vi "Notify Counter Branch.vi"(8 "EventLog":refnum<class "abs_EventLog.lvclass">, 9 "Time (ms)":u32=40, 10 "Blackboard Group":string="B", 11 "Blackboard in":refnum<class "Blackboard.lvclass">) -> (3 "bt_Node out":refnum<class "bt_Node.lvclass">)   [LabVIEW 2021]
uses:
  Blackboard/Blackboard.lvclass
  Support/Nodes/abs_Node/bt_Node.lvclass
  Support/Nodes/Decorators/Repeater/Support/Finish On - Type.ctl
  Blackboard/Blackboard.lvclass/Blackboard.ctl
  Support/Nodes/Leaves/abs_Type Leaf/abs_Type Leaf.lvclass/abs_Type Leaf.ctl
  Blackboard/Get Value Type/Get I32.vi
  Blackboard/Support/Index Group.vi
  Blackboard/Support/Index Tags.vi
  Support/Nodes/Leaves/abs_Type Leaf/Properties/Write Value Class.vi
  <vilib>/TSA/Abstract Data Classes/Abs_Types/I32 Integer/Abs_I32 Integer.lvclass
  C:/Program Files (x86)/National Instruments/LabVIEW 2021/vi.lib/TSA/Abstract Data Classes/Abs_Types/Value/Abs_Value.lvclass
  C:/Program Files (x86)/National Instruments/LabVIEW 2021/vi.lib/TSA/Abstract Data Classes/Abs_Types/Numeric/Abs_Numeric.lvclass
  <vilib>/TSA/Omni-Bus/Local Bus/Support/I32/Local Bus_I32.lvclass
  Support/Nodes/Leaves/Test Boolean/Test Abs_Boolean.lvclass
  C:/Users/timst/Documents/Repositories/LV_Behaviour_Tree/Source/Support/Nodes/abs_Node/bt_Node.lvclass
  C:/Users/timst/Documents/Repositories/LV_Behaviour_Tree/Source/Support/Nodes/Leaves/abs_Type Leaf/abs_Type Leaf.lvclass
  <vilib>/TSA/Abstract Data Classes/Abs_Types/Boolean/Abs_Boolean.lvclass
  C:/Program Files (x86)/National Instruments/LabVIEW 2021/vi.lib/TSA/Abstract Data Classes/Abs_Types/Type/Abs_Type.lvclass
  <vilib>/TSA/Omni-Bus/Local Bus/Support/Initialise DVR's.vi
  <vilib>/TSA/Abstract Data Classes/Abs_Types/Value/Abs_Value.lvclass
  <vilib>/TSA/Abstract Data Classes/Abs_Types/Type/Abs_Type.lvclass
  <vilib>/TSA/Omni-Bus/Local Bus/Support/DBL/Local Bus_DBL.lvclass
  <vilib>/TSA/Omni-Bus/Local Bus/Support/SGL/Local Bus_SGL.lvclass
  <vilib>/TSA/Omni-Bus/Local Bus/Support/EXT/Local Bus_EXT.lvclass
  <vilib>/TSA/Omni-Bus/Local Bus/Support/Bool/Local Bus_Boolean.lvclass
  <vilib>/TSA/Omni-Bus/Local Bus/Support/STR/Local Bus_String.lvclass
  <vilib>/TSA/Omni-Bus/Local Bus/Support/Variant/Local Bus_Variant.lvclass
  <vilib>/TSA/Omni-Bus/Local Bus/Support/WFM/Local Bus_Waveform.lvclass
  <vilib>/TSA/Omni-Bus/Local Bus/Support/Time/Local Bus_Time.lvclass
  <vilib>/TSA/Omni-Bus/Local Bus/Support/U8/Local Bus_U8.lvclass
  <vilib>/TSA/Omni-Bus/Local Bus/Support/U16/Local Bus_U16.lvclass
  <vilib>/TSA/Omni-Bus/Local Bus/Support/U32/Local Bus_U32.lvclass
  <vilib>/TSA/Omni-Bus/Local Bus/Support/U64/Local Bus_U64.lvclass
  <vilib>/TSA/Omni-Bus/Local Bus/Support/I8/Local Bus_I8.lvclass
  <vilib>/TSA/Omni-Bus/Local Bus/Support/I16/Local Bus_I16.lvclass
  <vilib>/TSA/Omni-Bus/Local Bus/Support/I64/Local Bus_I64.lvclass
  <vilib>/TSA/Omni-Bus/Local Bus/Support/CSGL/Local Bus_CSGL.lvclass
  <vilib>/TSA/Omni-Bus/Local Bus/Support/CDBL/Local Bus_CDBL.lvclass
  <vilib>/TSA/Omni-Bus/Local Bus/Support/CEXT/Local Bus_CEXT.lvclass
  <vilib>/TSA/Omni-Bus/Local Bus/Support/Type/Local Bus_Type.lvclass
  <vilib>/TSA/Abstract Data Classes/Functions/Compare/Support/Greater Equal/I32/Method.vi
  <vilib>/TSA/Abstract Data Classes/Functions/Math/Support/Increment/I32/Method.vi
  <vilib>/TSA/Abstract Data Classes/Constants/Support/I32/I32.vi
  BT.lvlib
  Support/Nodes/Decorators/Repeater/bt_Repeater.lvclass
  C:/Program Files (x86)/National Instruments/LabVIEW 2021/vi.lib/TSA/Abstract Data Classes/Abs_Types/Integer/Abs_Integer.lvclass
  C:/Program Files (x86)/National Instruments/LabVIEW 2021/vi.lib/TSA/Abstract Data Classes/Abs_Types/I32 Integer/Abs_I32 Integer.lvclass
  <vilib>/TSA/Abstract Data Classes/Functions/Compare/Support/Greater Equal/I32/Greater Equal_I32.lvclass
  <vilib>/TSA/Abstract Data Classes/Functions/Math/Support/Increment/I32/Increment_I32.lvclass
  <vilib>/TSA/Abstract Data Classes/Constants/Support/I32/Const_I32.lvclass
  <vilib>/TSA/Abstract Data Classes/Constants/Support/Str/Str.vi
  <vilib>/TSA/Abstract Data Classes/Constants/Support/Str/Const_Str.lvclass
  Support/Nodes/Leaves/Log/bt_Log.lvclass
  C:/Users/timst/Documents/Repositories/LV_Behaviour_Tree/Source/Support/Nodes/Leaves/Leaf/bt_Leaf.lvclass
  C:/Users/timst/Documents/Repositories/LV_Behaviour_Tree/Source/Support/Nodes/Leaves/Log/bt_Log.lvclass
  <vilib>/TSA/Event Log/abs_EventLog/abs_EventLog.lvclass
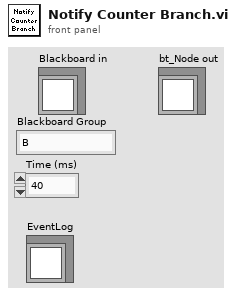
[diagram p1: front panel]
types:
  T1 = typedef "BT.lvlib/bt_Repeater.lvclass/Finish On - Type.ctl" = enum16{"Success", "Failure", "Never"}
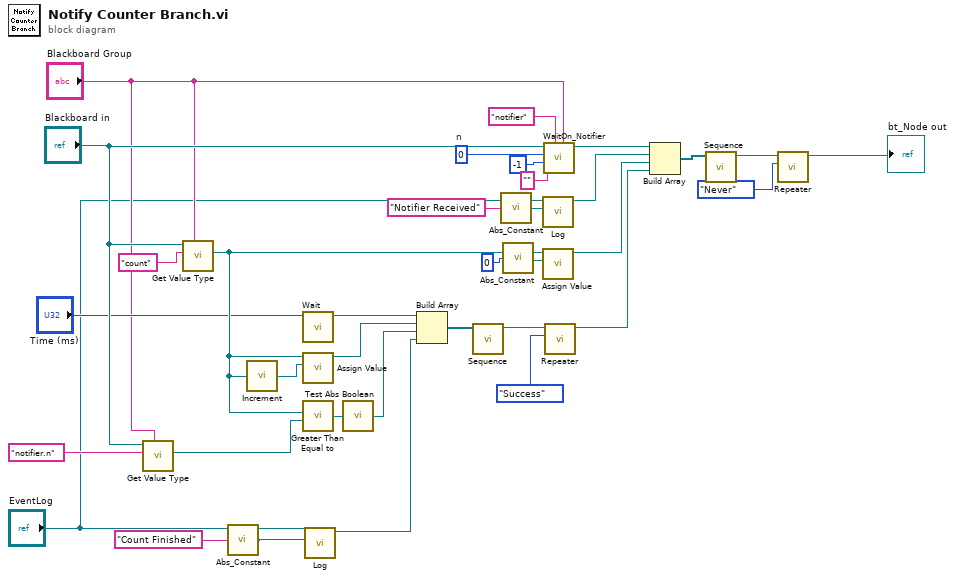
[diagram p0: block diagram]
diagram:
  w11 = 0  # n
  n1 = call-poly "Get Value Type.vi"("Tag Group"="Blackboard Group", "Tag"="notifier.n", "Blackboard in"="Blackboard in") -> ("Value"=w34:refnum<class "Abs_I32 Integer.lvclass">)  [unwired: 5 in, 3 out]
  n2 = call-poly "Get Value Type.vi"("Tag Group"="Blackboard Group", "Tag"="count", "Blackboard in"="Blackboard in") -> ("Value"=w33:refnum<class "Abs_I32 Integer.lvclass">)  [unwired: 5 in, 3 out]
  n3 = call-poly <vilib>:"Abs_Constant.vi"("String"="Count Finished") -> ("Abs_String.lvclass"=w2:refnum<class "Abs_String.lvclass">)  [unwired: 4 in]
  n4 = call-poly <vilib>:"Increment.vi"("Value"=w33) -> ("Result"=w19:refnum<class "Abs_I32 Integer.lvclass">)  [unwired: 4 in]
  n5 = call "Wait.vi"("Time (ms)"="Time (ms)") -> ("Node Out"=w14:refnum<class "bt_Node.lvclass">)  [unwired: 10 in]
  n6 = call "Assign Value.vi"("Assigned Value"=w19, "Value"=w33) -> ("Node Out"=w18:refnum<class "bt_Node.lvclass">)  [unwired: 9 in]
  n7 = call-poly <vilib>:"Greater Than Equal to.vi"("Value B"=w34, "Value A"=w33) -> ("Result"=w17:refnum<class "Abs_Boolean.lvclass">)  [unwired: 4 in]
  n8 = call "Log.vi"("Message"=w2, "EventLog"="EventLog") -> ("node out"=w6:refnum<class "bt_Log.lvclass">)  [unwired: 9 in]
  n9 = call "Test Abs Boolean.vi"("Abs_Boolean.lvclass"=w17) -> ("abs_Node"=w16:refnum<class "bt_Node.lvclass">)  [unwired: 4 in]
  n10 = Build Array(w14, w18, w16, w6) -> (w24:refnum<class "bt_Node.lvclass">[])
  n11 = call "Sequence.vi"("Nodes"=w24) -> ("Node"=w25:refnum<class "bt_Node.lvclass">)  [unwired: 10 in]
  n12 = call-poly <vilib>:"Abs_Constant.vi"("String"="Notifier Received") -> ("Abs_String.lvclass"=w5:refnum<class "Abs_String.lvclass">)  [unwired: 4 in]
  n13 = call-poly <vilib>:"Abs_Constant.vi"("Value"=0 ("n")) -> ("Constant"=w20:refnum<class "Abs_I32 Integer.lvclass">)  [unwired: 4 in]
  n14 = call "Log.vi"("Message"=w5, "EventLog"="EventLog") -> ("node out"=w7:refnum<class "bt_Log.lvclass">)  [unwired: 9 in]
  n15 = call "Assign Value.vi"("Assigned Value"=w20, "Value"=w33) -> ("Node Out"=w15:refnum<class "bt_Node.lvclass">)  [unwired: 9 in]
  n16 = call "WaitOn_Notifier.vi"("Blackboard Group"="Blackboard Group", "Notifier Name"="notifier" ("Name"), "Tag Root"="", "Timeout (ms)"=-1, "Message Type"=w11, "bt_Blackboard in"="Blackboard in") -> ("Node Out"=w10:refnum<class "bt_Node.lvclass">)  [unwired: 4 in, 1 out]
  n17 = call "Repeater.vi"("Finish On"=Finish_On_-_Type."Success", "Node In"=w25) -> ("Node Out"=w26:refnum<class "bt_Node.lvclass">)  [unwired: 9 in]
  n18 = Build Array(w10, w7, w15, w26) -> (w28:refnum<class "bt_Node.lvclass">[])
  n19 = call "Sequence.vi"("Nodes"=w28) -> ("Node"=w27:refnum<class "bt_Node.lvclass">)  [unwired: 10 in]
  n20 = call "Repeater.vi"("Finish On"=Finish_On_-_Type."Never", "Node In"=w27) -> ("Node Out"=→"bt_Node out":refnum<class "bt_Node.lvclass">)  [unwired: 9 in]
